vi "DPOAE Raw Waveform Test.vi"() -> ()   [LabVIEW 2020]
uses:
  Typedefs/DP-DataAcq.ctl
  Typedefs/DP-Freqs.ctl
  Utility VIs/Comparison VIs/Approx Equal (1D-Scalar).vi
  Utility VIs/Math VIs/FFT x(t) to dB,Degrees (1D).vi
panel:
  out "Output Array":dbl[](array[numeric])
  out "Waveform Graph 2":dbl[](graph)
  in  "Mic Gain (dB)":dbl=40.0
  out "Waveform Graph":dbl[](graph)
  out "index of element":i32
  in  "L2":dbl=50.0
  in  "F2":dbl=12000.0
  out "Data matrix":dbl[][](array[numeric])=[[10.0, 26660.0, 32000.0, 19.87, 17.15, 4.28, 4.43, -11.58, -11.88, 0.0, nan], [15.0, 26660.0, 32000.0, 25.26, 12.82, 5.74, 4.53, -10.76, -11.66, 0.0, nan], [20.0, 26660.0, 32000.0, 30.19, 20.84, 7.69, 4.48, -14.28, -11.15, 0.0, nan], [25.0, 26660.0, 32000.0, 35.28, 25.61, 3.66, 5.97, -8.88, -11.6, 0.0, nan], [30.0, 26660.0, 32000.0, 40.25, 29.95, 4.82, 5.16, -14.39, -13.03, 0.0, nan], [35.0, 26660.0, 32000.0, 45.24, 35.29, 7.06, 6.06, -11.69, -12.64, 0.0, nan], [40.0, 26660.0, 32000.0, 50.27, 40.32, 8.83, 5.15, -8.47, -13.37, 0.0, nan], [45.0, 26660.0, 32000.0, 55.27, 45.04, 15.76, 5.91, -8.83, -11.07, 0.0, nan], [50.0, 26660.0, 32000.0, 60.3, 50.15, 18.46, 6.69, -15.27, -11.44, 0.0, nan], [55.0, 26660.0, 32000.0, 65.34, 55.15, 18.51, 5.1, -7.72, -13.75, 0.0, nan], [60.0, 26660.0, 32000.0, 70.39, 60.07, 18.72, 5.48, -10.97, -12.6, 0.0, nan], [65.0, 26660.0, 32000.0, 75.4, 65.14, 20.86, 6.2, -14.21, -12.75, 0.0, nan], [70.0, 26660.0, 32000.0, 80.41, 70.13, 19.74, 7.97, -13.01, -13.31, 0.0, nan], [75.0, 26660.0, 32000.0, 85.34, 75.13, 16.8, 4.2, -10.39, -11.78, 0.0, nan], [80.0, 26660.0, 32000.0, 90.05, 80.19, 24.41, 5.51, -3.93, -10.58, 0.0, nan], [10.0, 20000.0, 24000.0, 19.69, 10.61, -2.79, -3.65, -16.43, -19.07, 0.0, nan], [15.0, 20000.0, 24000.0, 24.79, 15.96, -5.32, -5.49, -25.48, -20.47, 0.0, nan], [20.0, 20000.0, 24000.0, 30.16, 19.7, -2.47, -4.93, -13.81, -20.34, 0.0, nan], [25.0, 20000.0, 24000.0, 35.09, 24.76, -3.83, -4.71, -17.75, -17.93, 0.0, nan], [30.0, 20000.0, 24000.0, 40.1, 30.08, -7.62, -4.7, -21.56, -19.04, 0.0, nan], [35.0, 20000.0, 24000.0, 45.11, 34.98, -7.37, -6.25, -15.13, -17.48, 0.0, nan], [40.0, 20000.0, 24000.0, 50.13, 39.94, -0.9, -3.77, -14.28, -19.51, 0.0, nan], [45.0, 20000.0, 24000.0, 55.13, 45.06, 2.55, -5.61, -9.19, -20.02, 0.0, nan], [50.0, 20000.0, 24000.0, 60.14, 50.05, 8.2, -3.28, -13.51, -21.52, 0.0, nan], [55.0, 20000.0, 24000.0, 65.11, 55.05, 13.29, -4.95, -5.44, -18.61, 0.0, nan], [60.0, 20000.0, 24000.0, 70.11, 60.05, 16.27, -7.23, -6.41, -20.82, 0.0, nan], [65.0, 20000.0, 24000.0, 75.08, 65.06, 17.69, -3.9, -5.45, -19.19, 0.0, nan], [70.0, 20000.0, 24000.0, 80.06, 69.97, 18.41, -5.29, -7.08, -20.31, 0.0, nan], [75.0, 20000.0, 24000.0, 85.12, 75.0, 16.35, -3.17, -6.81, -18.78, 0.0, nan], [80.0, 20000.0, 24000.0, 89.89, 79.99, 20.08, -5.34, -8.45, -17.82, 0.0, nan], [10.0, 13340.0, 16000.0, 20.19, 10.03, -24.5, -17.49, -26.94, -19.74, 0.0, nan], [15.0, 13340.0, 16000.0, 24.94, 14.85, -19.66, -19.46, -17.17, -20.55, 0.0, nan], [20.0, 13340.0, 16000.0, 29.89, 19.8, -16.74, -19.65, -17.16, -17.4, 0.0, nan], [25.0, 13340.0, 16000.0, 34.93, 24.75, -17.03, -19.73, -23.83, -21.42, 0.0, nan], [30.0, 13340.0, 16000.0, 39.96, 29.97, -10.4, -17.41, -16.43, -20.08, 0.0, nan], [35.0, 13340.0, 16000.0, 44.97, 34.89, -4.28, -19.13, -21.76, -20.14, 0.0, nan], [40.0, 13340.0, 16000.0, 49.97, 39.97, 4.15, -19.74, -21.75, -18.1, 0.0, nan], [45.0, 13340.0, 16000.0, 54.99, 44.99, 10.11, -17.79, -23.65, -20.42, 0.0, nan], [50.0, 13340.0, 16000.0, 59.99, 49.99, 15.0, -19.65, -14.97, -18.13, 0.0, nan], [55.0, 13340.0, 16000.0, 64.98, 54.99, 18.58, -18.9, -11.32, -14.18, 0.0, nan], [60.0, 13340.0, 16000.0, 69.99, 59.98, 20.42, -18.13, -4.53, -17.47, 0.0, nan], [65.0, 13340.0, 16000.0, 74.99, 64.96, 20.6, -19.69, -1.98, -19.0, 0.0, nan], [70.0, 13340.0, 16000.0, 80.0, 69.95, 16.52, -19.64, -0.59, -19.4, 0.0, nan], [75.0, 13340.0, 16000.0, 85.0, 74.94, 25.55, -20.53, 0.25, -20.79, 0.0, nan], [80.0, 13340.0, 16000.0, 89.99, 79.94, 35.67, -20.59, 11.29, -20.1, 0.0, nan], [10.0, 10000.0, 12000.0, 20.05, 10.04, -9.99, -11.88, -9.79, -10.63, 0.0, nan], [15.0, 10000.0, 12000.0, 25.1, 15.12, -8.89, -9.88, -9.06, -8.58, 0.0, nan], [20.0, 10000.0, 12000.0, 30.01, 19.89, -0.43, -10.0, -2.83, -11.58, 0.0, nan], [25.0, 10000.0, 12000.0, 34.94, 25.03, 7.47, -9.01, 0.56, -9.96, 0.0, nan], [30.0, 10000.0, 12000.0, 39.92, 29.88, 13.88, -11.05, 2.67, -10.85, 0.0, nan], [35.0, 10000.0, 12000.0, 44.92, 34.93, 20.91, -11.2, 5.85, -10.02, 0.0, nan], [40.0, 10000.0, 12000.0, 49.91, 39.95, 26.39, -11.14, 6.15, -11.07, 0.0, nan], [45.0, 10000.0, 12000.0, 54.97, 44.95, 31.34, -11.1, 4.85, -12.38, 0.0, nan], [50.0, 10000.0, 12000.0, 59.97, 49.98, 34.94, -10.34, 1.89, -11.49, 0.0, nan], [55.0, 10000.0, 12000.0, 64.95, 54.98, 36.43, -10.15, 6.84, -10.66, 0.0, nan], [60.0, 10000.0, 12000.0, 69.92, 59.98, 33.68, -9.73, 15.91, -10.25, 0.0, nan], [65.0, 10000.0, 12000.0, 74.89, 64.98, 34.29, -7.64, 21.22, -9.99, 0.0, nan], [70.0, 10000.0, 12000.0, 79.93, 70.0, 47.98, -10.49, 24.72, -8.44, 0.0, nan], [75.0, 10000.0, 12000.0, 84.98, 75.06, 53.77, -10.62, 29.52, -11.35, 0.0, nan], [80.0, 10000.0, 12000.0, 90.0, 80.1, 57.16, -9.01, 35.4, -9.81, 0.0, nan], [10.0, 6660.0, 8000.0, 19.92, 10.89, -11.9, -14.0, -15.14, -11.64, 0.0, nan], [15.0, 6660.0, 8000.0, 24.75, 15.52, -9.13, -13.55, -10.22, -13.4, 0.0, nan], [20.0, 6660.0, 8000.0, 29.7, 20.18, -13.01, -13.02, -14.8, -11.36, 0.0, nan], [25.0, 6660.0, 8000.0, 34.73, 25.2, -13.99, -11.24, -8.65, -11.93, 0.0, nan], [30.0, 6660.0, 8000.0, 39.72, 30.24, -6.67, -12.22, -11.91, -14.3, 0.0, nan], [35.0, 6660.0, 8000.0, 44.82, 35.27, 0.21, -13.43, -9.8, -14.5, 0.0, nan], [40.0, 6660.0, 8000.0, 49.84, 40.26, 9.14, -13.26, -4.24, -13.09, 0.0, nan], [45.0, 6660.0, 8000.0, 54.91, 45.29, 15.11, -12.52, -3.14, -12.44, 0.0, nan], [50.0, 6660.0, 8000.0, 59.9, 50.18, 20.55, -12.04, -1.34, -13.17, 0.0, nan], [55.0, 6660.0, 8000.0, 64.96, 55.14, 22.71, -12.3, -5.8, -12.57, 0.0, nan], [60.0, 6660.0, 8000.0, 69.88, 60.0, 24.28, -9.98, -3.59, -14.8, 0.0, nan], [65.0, 6660.0, 8000.0, 74.92, 65.03, 21.21, -11.17, 9.87, -12.1, 0.0, nan], [70.0, 6660.0, 8000.0, 79.89, 69.96, 22.62, -11.49, 17.15, -13.6, 0.0, nan], [75.0, 6660.0, 8000.0, 84.87, 74.92, 34.03, -12.34, 22.11, -13.25, 0.0, nan], [80.0, 6660.0, 8000.0, 89.96, 80.03, 39.33, -12.68, 30.2, -11.26, 0.0, nan], [10.0, 4660.0, 5600.0, 19.91, 9.58, -20.83, -25.32, -13.78, -5.94, 0.0, nan], [15.0, 4660.0, 5600.0, 25.03, 14.56, -19.37, -22.35, -8.99, -5.79, 0.0, nan], [20.0, 4660.0, 5600.0, 29.82, 19.86, -19.17, -21.11, -7.0, -4.89, 0.0, nan], [25.0, 4660.0, 5600.0, 34.91, 24.83, -20.64, -22.18, -11.84, -5.64, 0.0, nan], [30.0, 4660.0, 5600.0, 39.86, 29.92, -13.23, -23.0, -5.06, -6.56, 0.0, nan], [35.0, 4660.0, 5600.0, 45.03, 34.8, -6.83, -21.26, -4.27, -6.35, 0.0, nan], [40.0, 4660.0, 5600.0, 49.89, 39.86, 1.68, -22.62, -0.44, -5.81, 0.0, nan], [45.0, 4660.0, 5600.0, 54.89, 44.87, 6.86, -21.59, 3.18, -5.77, 0.0, nan], [50.0, 4660.0, 5600.0, 60.07, 49.8, 7.67, -19.71, 0.49, -9.26, 0.0, nan], [55.0, 4660.0, 5600.0, 64.91, 54.85, 8.22, -23.75, -1.76, -7.04, 0.0, nan], [60.0, 4660.0, 5600.0, 69.93, 59.83, 12.8, -21.69, 8.82, -4.39, 0.0, nan], [65.0, 4660.0, 5600.0, 74.97, 64.77, 22.51, -22.13, 15.08, -4.79, 0.0, nan], [70.0, 4660.0, 5600.0, 80.04, 69.81, 29.07, -23.05, 19.21, -6.05, 0.0, nan], [75.0, 4660.0, 5600.0, 85.12, 74.77, 29.31, -18.69, 27.73, -4.62, 0.0, nan], [80.0, 4660.0, 5600.0, 90.11, 79.77, 29.68, -21.88, 37.68, -6.52, 0.0, nan], [10.0, 3340.0, 4000.0, 20.21, 10.39, -22.35, -20.26, -6.56, -6.11, 0.0, nan], [15.0, 3340.0, 4000.0, 25.3, 15.3, -24.7, -18.85, -8.71, -7.41, 0.0, nan], [20.0, 3340.0, 4000.0, 30.14, 20.23, -18.49, -19.55, -3.69, -8.01, 0.0, nan], [25.0, 3340.0, 4000.0, 35.24, 25.21, -5.82, -20.43, -3.71, -7.59, 0.0, nan], [30.0, 3340.0, 4000.0, 40.13, 30.13, 0.59, -20.96, -5.78, -5.89, 0.0, nan], [35.0, 3340.0, 4000.0, 45.03, 35.11, 5.26, -20.72, -0.04, -8.49, 0.0, nan], [40.0, 3340.0, 4000.0, 50.0, 40.16, 8.36, -20.97, 4.07, -5.09, 0.0, nan], [45.0, 3340.0, 4000.0, 55.04, 45.11, 10.93, -20.28, 2.57, 1.51, 0.0, nan], [50.0, 3340.0, 4000.0, 60.03, 50.11, 6.63, -11.11, 0.01, -4.6, 0.0, nan], [55.0, 3340.0, 4000.0, 64.91, 55.11, 15.87, -17.64, 9.46, -6.63, 0.0, nan], [60.0, 3340.0, 4000.0, 69.85, 60.05, 27.11, -16.28, 19.54, -6.51, 0.0, nan], [65.0, 3340.0, 4000.0, 74.94, 65.05, 32.91, -13.0, 29.01, -4.21, 0.0, nan], [70.0, 3340.0, 4000.0, 79.94, 70.06, 27.71, -17.12, 39.65, -1.84, 0.0, nan], [75.0, 3340.0, 4000.0, 85.06, 75.08, 30.16, -18.36, 49.77, -7.98, 0.0, nan], [80.0, 3340.0, 4000.0, 90.05, 79.98, 35.46, -16.89, 60.32, 1.18, 0.0, nan], [10.0, 2320.0, 2780.0, 20.0, 10.44, -14.73, -11.76, -2.5, -6.58, 0.0, nan], [15.0, 2320.0, 2780.0, 24.93, 15.3, -11.66, -14.39, -8.94, -14.48, 0.0, nan], [20.0, 2320.0, 2780.0, 29.95, 20.28, -13.2, -13.33, -10.99, -14.33, 0.0, nan], [25.0, 2320.0, 2780.0, 34.98, 25.32, -12.87, -11.02, -10.9, -13.06, 0.0, nan], [30.0, 2320.0, 2780.0, 40.03, 30.42, -11.25, -14.54, -13.59, -13.57, 0.0, nan], [35.0, 2320.0, 2780.0, 45.04, 35.3, -8.93, -11.45, -14.97, -12.37, 0.0, nan], [40.0, 2320.0, 2780.0, 50.11, 40.33, -2.39, -12.1, 3.43, -4.58, 0.0, nan], [45.0, 2320.0, 2780.0, 55.11, 45.28, 4.52, -12.66, -4.8, -7.27, 0.0, nan], [50.0, 2320.0, 2780.0, 60.15, 50.29, 9.38, -12.14, -2.73, -12.96, 0.0, nan], [55.0, 2320.0, 2780.0, 65.1, 55.19, 13.57, -12.59, 1.8, -6.28, 0.0, nan], [60.0, 2320.0, 2780.0, 70.15, 60.24, 20.57, -9.89, 11.45, -11.87, 0.0, nan], [65.0, 2320.0, 2780.0, 75.17, 65.27, 25.89, -8.47, 20.75, -12.88, 0.0, nan], [70.0, 2320.0, 2780.0, 80.19, 70.31, 33.52, -6.41, 30.34, -14.44, 0.0, nan], [75.0, 2320.0, 2780.0, 85.17, 75.26, 34.71, -0.34, 40.02, -9.21, 0.0, nan], [80.0, 2320.0, 2780.0, 90.16, 80.2, 31.33, -1.31, 49.99, -9.75, 0.0, nan]]
  in  "Data file":path=path "C:/Data/XYZ DATA/XYZ998/DP-149-2"
  in  "Probe Tube Cal":path=path "C:/Data/XYZ DATA/XYZ998/guinea_pig_ProbeTube.calib"
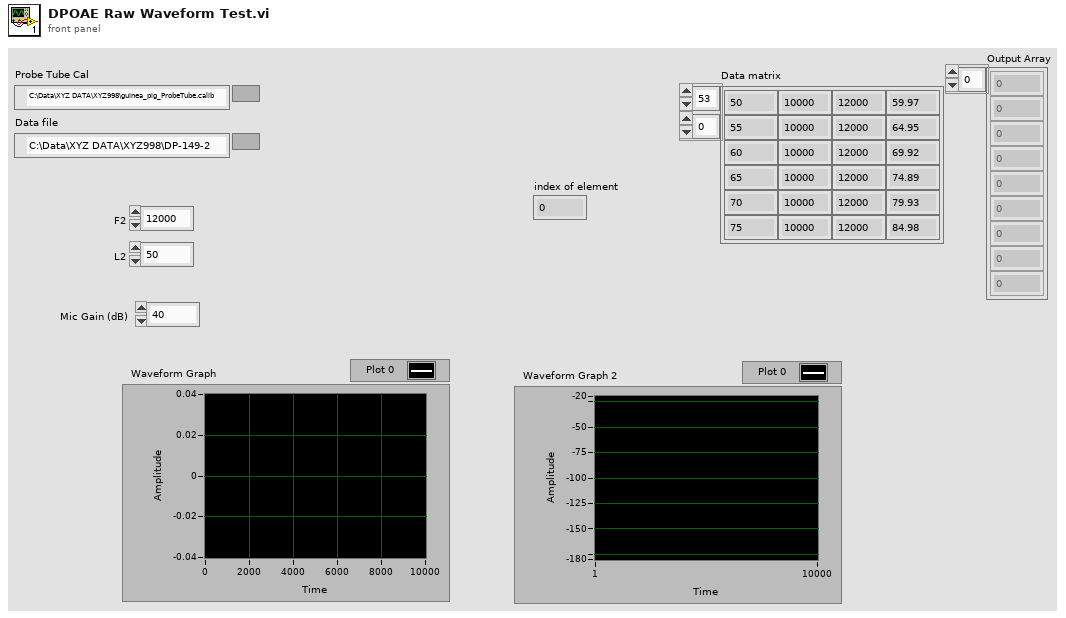
[diagram p1: front panel]
types:
  T1 = typedef "DP-Freqs.ctl" = cluster{"f1":dbl, "f2":dbl, "2f1-f2":dbl}
  T2 = typedef "DP-DataAcq.ctl" = cluster{"#spectra avgs":i32[], "#time avgs":i32[], "dt (ms)":dbl, "df (kHz)":dbl, "Npts":i32, "Save waves?":bool, "Data File":path, "AI Channels":u16[], "Sampling rate (Hz)":dbl, "Probe Tube Sensitivity":cluster{"Frequency":dbl[], "Mag":dbl[]}, "Mic gain (dB)":dbl, "ptIndex":i32}
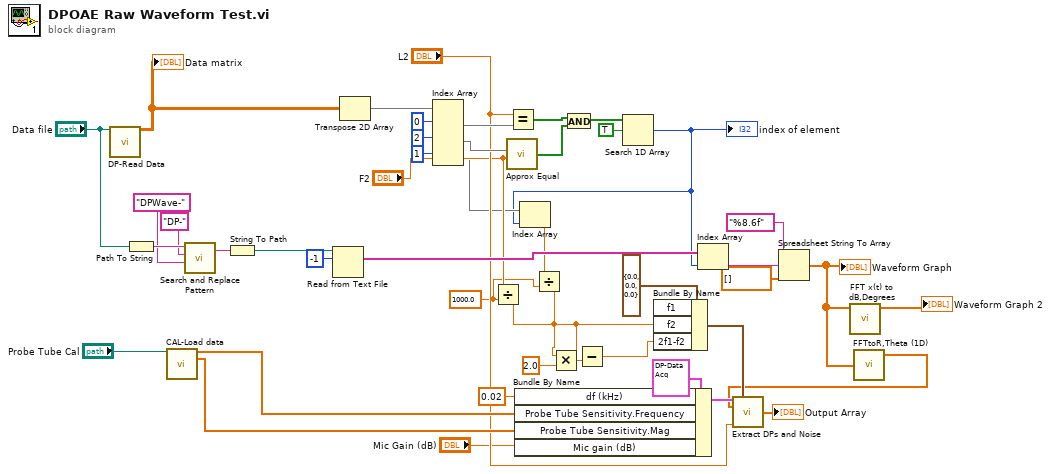
[diagram p0: block diagram]
diagram:
  w1 = 1000.0 ("y")
  n1 = call "DP-Read Data.vi"("Path"="Data file") -> ("Data matrix"=w41:dbl[][])  [unwired: 11 in, 3 out]
  "Data matrix" <- w41
  n2 = Path To String(path="Data file") -> (string=w46:string)
  n3 = call "CAL-Load data.vi"("user path"="Probe Tube Cal") -> ("Frequency (Hz)"=w22:dbl[], "Mag"=w21:dbl[])  [unwired: 7 in, 6 out]
  n4 = call <vilib>:"Search and Replace Pattern.vi"("string"=w46, "regular expression (\"\")"="DP-" ("regular expression (\"\")"), "replace string (\"\")"="DPWave-" ("regular expression (\"\")")) -> ("result string"=w43:string)  [unwired: 2 in, 1 out]
  n5 = String To Path(string=w43) -> (path=w31:path)
  n6 = Read from Text File(file (use dialog)=w31, count=-1) -> (text=w29:string[])  [unwired: 2 in, 3 out]
  n7 = Transpose 2D Array(2D array=w41) -> (transposed array=w40:dbl[][])
  n8 = Index Array(array=w40, index (row) #1=0 ("index (row)"), index (row) #2=2 ("index (row)"), index (row) #3=1 ("index (row)")) -> (element #1=w39:dbl[], element #2=w38:dbl[], element #3=w5:dbl[])  [unwired: 3 in]
  n9 = Divide(x="F2", y=w1) -> (x/y=w7:dbl)
  n10 = call-poly "Approx Equal.vi"("Y"="F2", "X"=w38) -> ("X approx Y?"=w36:bool[])  [unwired: 4 in]
  n11 = Equal?(x="L2", y=w39) -> (x = y?=w37:bool[])
  n12 = Bundle By Name(cluster=T2 {"#spectra avgs"=[], "#time avgs"=[], "dt (ms)"=0.0, "df (kHz)"=0.0, "Npts"=0, "Save waves?"=FALSE, "Data File"=path "", "AI Channels"=[], "Sampling rate (Hz)"=0.0, "Probe Tube Sensitivity"={"Frequency"=[], "Mag"=[]}, "Mic gain (dB)"=0.0, "ptIndex"=0} ("DataAcq"), "df (kHz)"=0.02, "Probe Tube Sensitivity.Frequency"=w22, "Probe Tube Sensitivity.Mag"=w21, "Mic gain (dB)"="Mic Gain (dB)") -> (w23:T2)
  n13 = And(x=w37, y=w36) -> (x .and. y?=w35:bool[])
  n14 = Search 1D Array(1D array=w35, element=TRUE) -> (index of element=w4:i32)  [unwired: 1 in]
  "index of element" <- w4
  n15 = Index Array(array=w5, index=w4) -> (element=w3:dbl)
  n16 = Divide(x=w3, y=w1) -> (x/y=w2:dbl)
  n17 = Multiply(x=w2, y=2.0) -> (x*y=w15:dbl)
  n18 = Subtract(x=w15, y=w7) -> (x-y=w9:dbl)
  n19 = Bundle By Name(cluster=T1 {"f1"=0.0, "f2"=0.0, "2f1-f2"=0.0} ("DP Freqs"), "f1"=w2, "f2"=w7, "2f1-f2"=w9) -> (w19:T1)
  n20 = Index Array(array=w29, index=w4) -> (element=w28:string)
  n21 = Spreadsheet String To Array(format string="%8.6f", spreadsheet string=w28, array type (2D Dbl)=dbl[] []) -> (array=w12:dbl[])  [unwired: 1 in]
  "Waveform Graph" <- w12
  n22 = call-poly "FFT x(t) to dB,Degrees.vi"("X"=w12) -> ("+Freq. Mag of FFT (dB rms)"=→"Waveform Graph 2":dbl[])  [unwired: 8 in, 2 out]
  n23 = call "FFTtoR,Theta (1D).VI"("X"=w12) -> ("+Freq. Mag of FFT"=w11:dbl[])  [unwired: 1 in, 1 out]
  n24 = call "Extract DPs and Noise.vi"("DataAcq"=w23, "DP Freqs"=w19, "Spectrum in Vrms"=w11, "SPL"="L2") -> ("Output Array"=→"Output Array":dbl[])  [unwired: 11 in]
